vi "全局变量：数据点个数.vi"() -> ()   [LabVIEW 2018]
panel:
  in  "数据点个数":i32
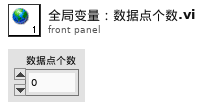
[diagram p1: front panel]
diagram:
